vi "RunVis.vi"(6 "Re-Init":bool, 7 "Index":i8, 8 "dt":i8, 9 "HMI to Control":T1, 10 "SensorInputData":T5, 11 "arguments":string[](array[string])) -> (1 "Done":bool, 2 "HMI to Control Out":T1, 3 "SensorInputDataOut":T5)   [LabVIEW 2015]
uses:
  Typedefs/Arm States.ctl
  Typedefs/IntakeWheelSenseOrManual.ctl
  Typedefs/ClawStates.ctl
  Typedefs/HMI_to_Control.ctl
  Typedefs/SensorInputData.ctl
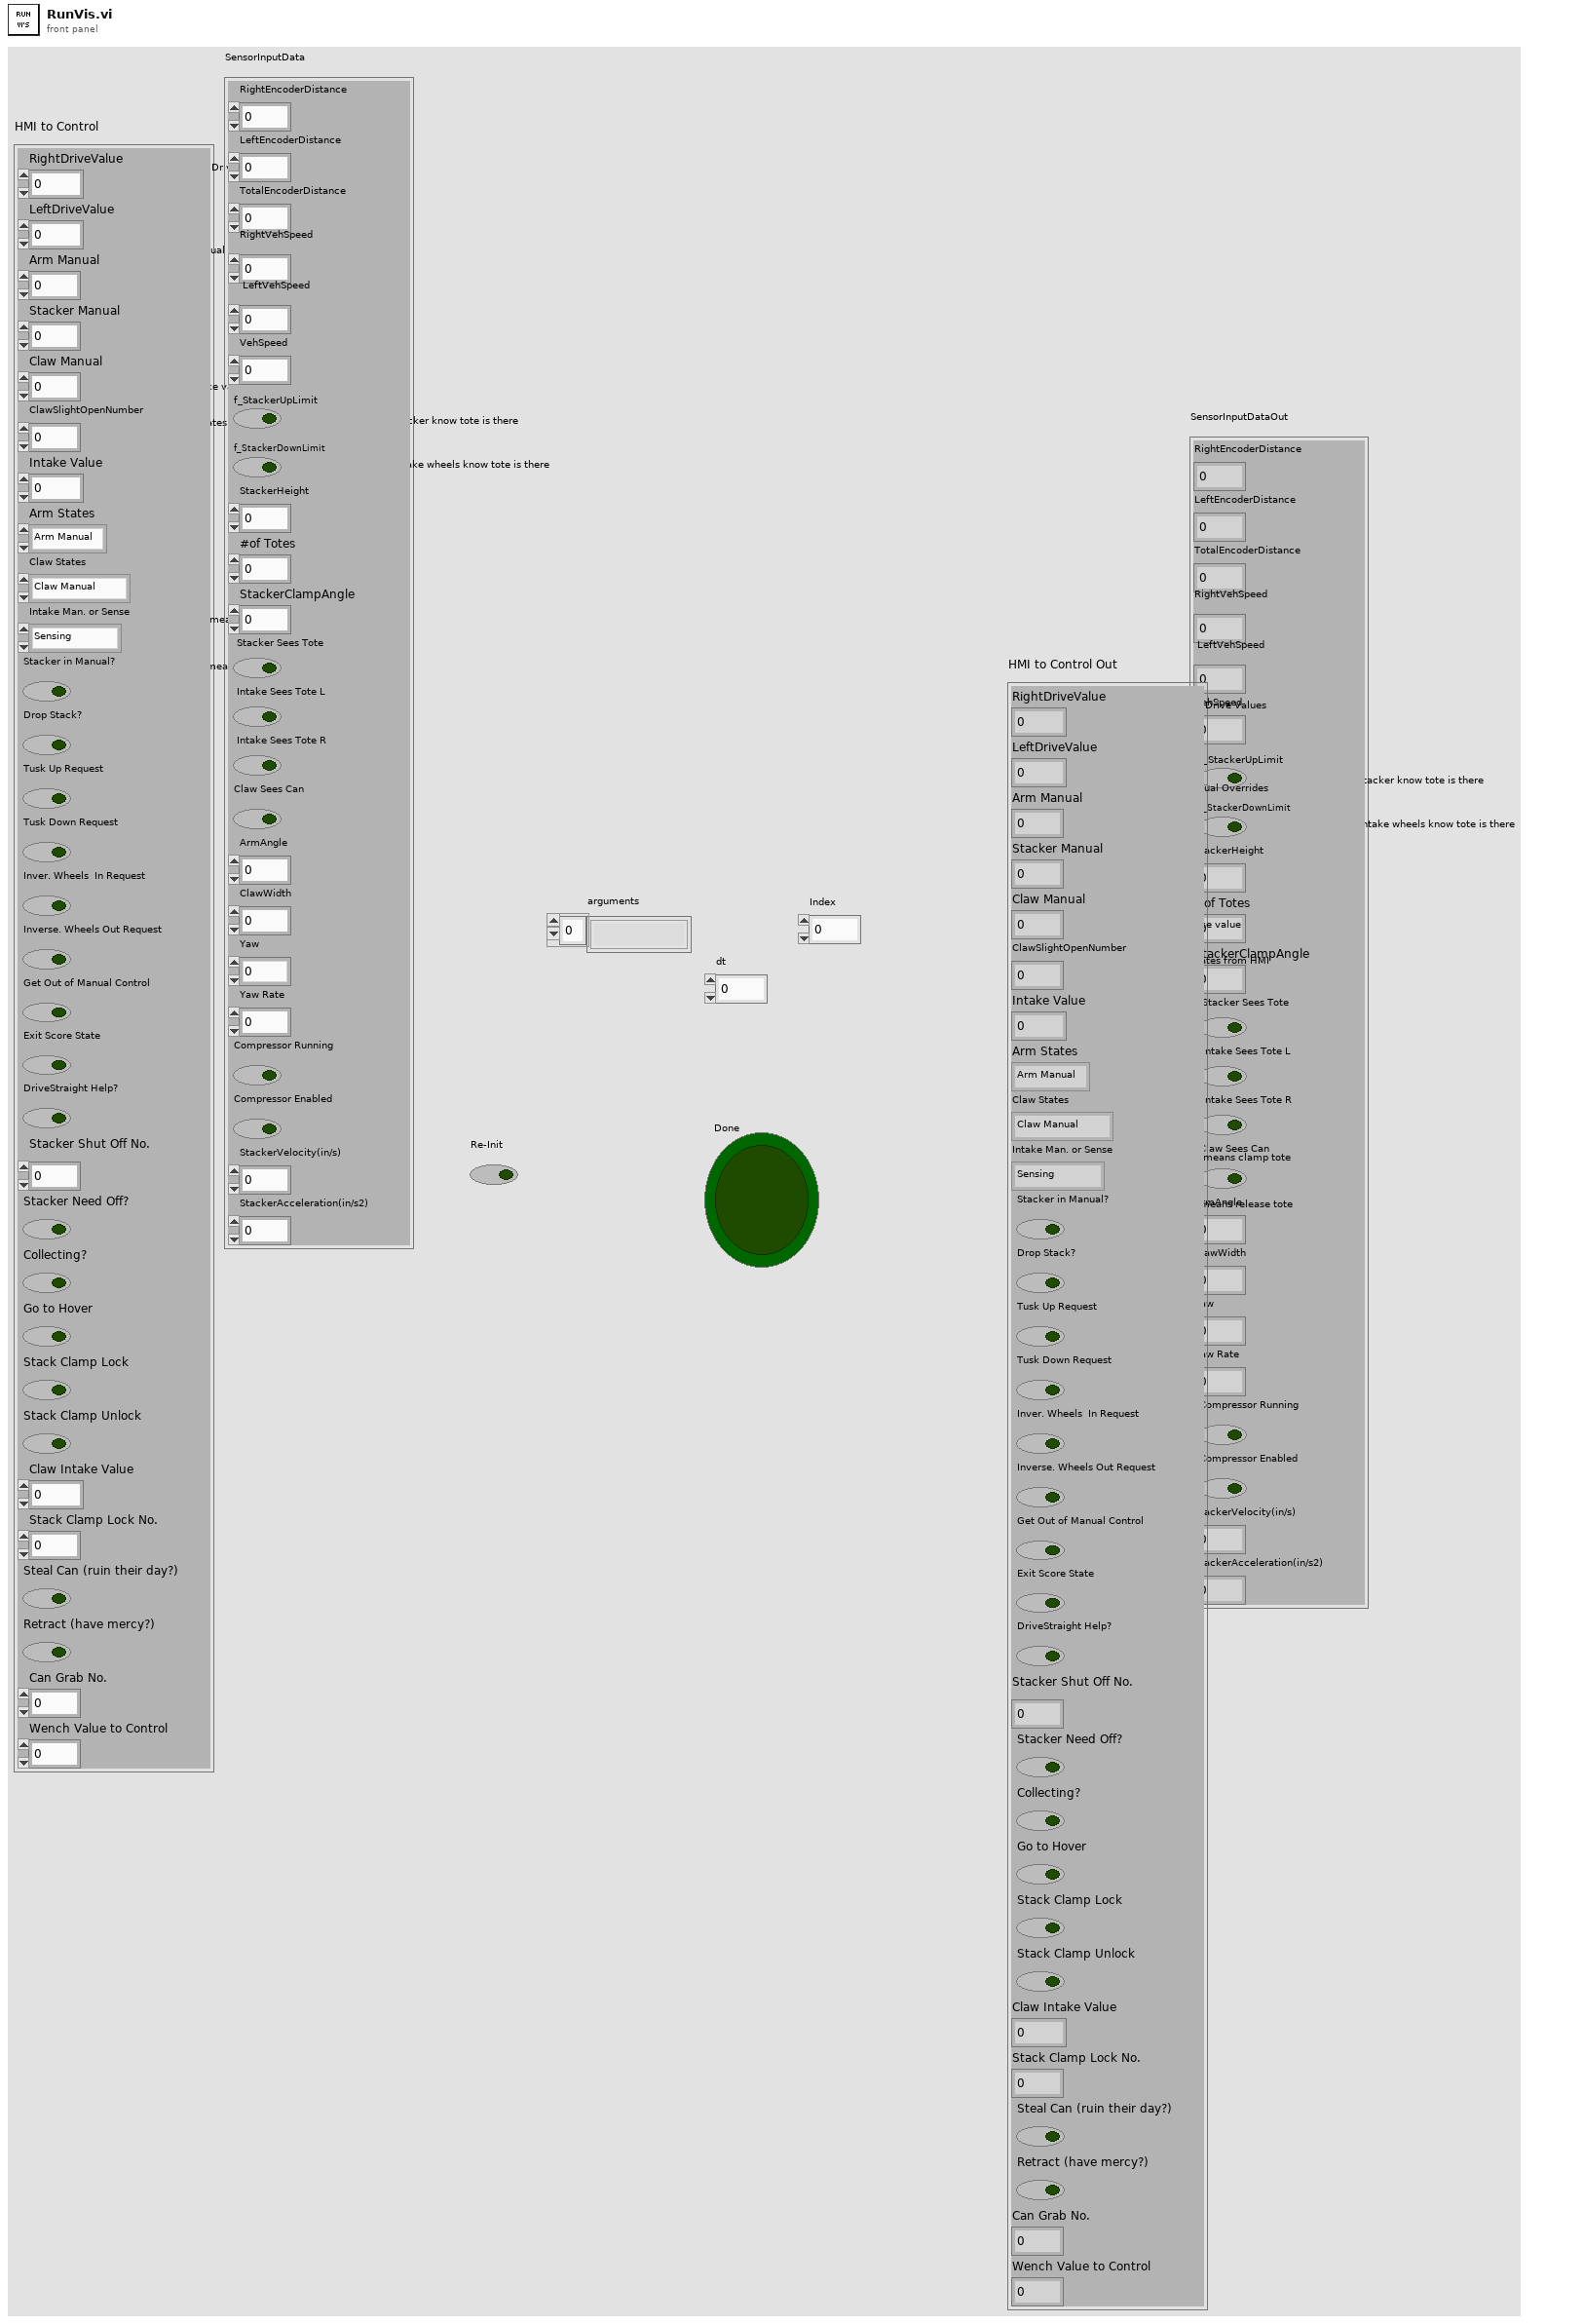
[diagram p1: front panel]
types:
  T1 = typedef "HMI_to_Control.ctl" = cluster{"RightDriveValue":dbl, "LeftDriveValue":dbl, "Arm Manual ":dbl, "Stacker Manual ":dbl, "Claw Manual ":dbl, "ClawSlightOpenNumber":i8, "Intake Value ":sgl, "Arm States":T2, "Claw States":T3, "Intake Man. or Sense":T4, "Stacker in Manual?":bool, "Drop Stack? ":bool, "Tusk Up Request":bool, "Tusk Down Request":bool, "Inver. Wheels  In Request":bool, "Inverse. Wheels Out Request ":bool, "Get Out of Manual Control":bool, "Exit Score State":bool, "DriveStraight Help?":bool, "Stacker Shut Off No.":i8, "Stacker Need Off?":bool, "Collecting?":bool, "Go to Hover":bool, "Stack Clamp Lock ":bool, "Stack Clamp Unlock ":bool, "Claw Intake Value ":sgl, "Stack Clamp Lock No. ":i8, "Steal Can (ruin their day?)":bool, "Retract (have mercy?)":bool, "Can Grab No. ":i8, "Wench Value to Control ":dbl}
  T2 = typedef "Arm States.ctl" = enum16{"Arm Manual ", "Ground", "Step", "1 Tote", "2 Tote", "3 Tote", "4 Tote", "5 Tote", "6 Tote", "Flip Can Arm", "Grab Can in auto", "Nudge"}
  T3 = typedef "ClawStates.ctl" = enum16{"Claw Manual ", "Claw Open", "Claw Closed", "Claw Slight Open", "Flip Can"}
  T4 = typedef "IntakeWheelSenseOrManual.ctl" = enum16{"Sensing", "Manual "}
  T5 = typedef "SensorInputData.ctl" = cluster{"RightEncoderDistance":dbl, "LeftEncoderDistance":dbl, "TotalEncoderDistance":dbl, "RightVehSpeed":dbl, "LeftVehSpeed":dbl, "VehSpeed":dbl, "f_StackerUpLimit":bool, "f_StackerDownLimit":bool, "StackerHeight":dbl, "#of Totes":u8, "StackerClampAngle":dbl, "Stacker Sees Tote":bool, "Intake Sees Tote L":bool, "Intake Sees Tote R":bool, "Claw Sees Can":bool, "ArmAngle":dbl, "ClawWidth":dbl, "Yaw":dbl, "Yaw Rate":dbl, "Compressor Running":bool, "Compressor Enabled":bool, "StackerVelocity(in/s)":dbl, "StackerAcceleration(in/s2)":dbl}
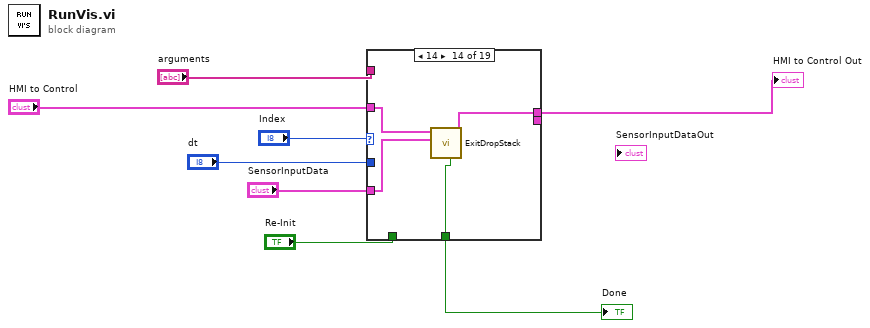
[diagram p0: block diagram]
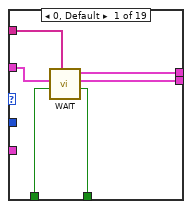
[diagram p2: hidden frame]
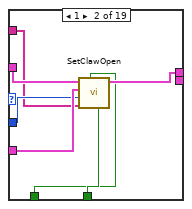
[diagram p3: hidden frame]
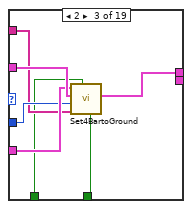
[diagram p4: hidden frame]
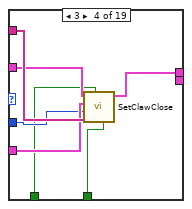
[diagram p5: hidden frame]
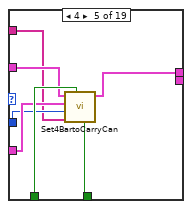
[diagram p6: hidden frame]
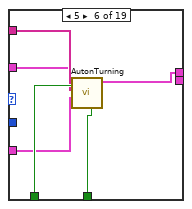
[diagram p7: hidden frame]
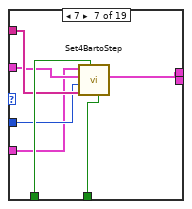
[diagram p8: hidden frame]
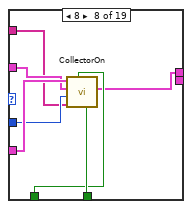
[diagram p9: hidden frame]
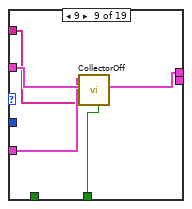
[diagram p10: hidden frame]
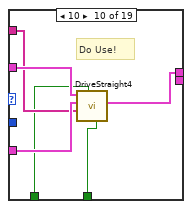
[diagram p11: hidden frame]
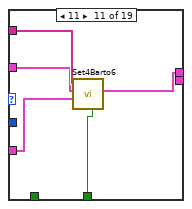
[diagram p12: hidden frame]
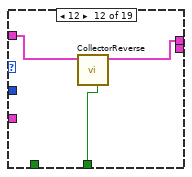
[diagram p13: hidden frame]
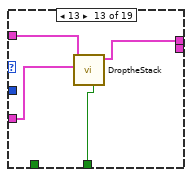
[diagram p14: hidden frame]
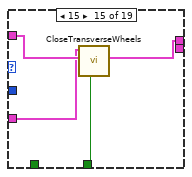
[diagram p15: hidden frame]
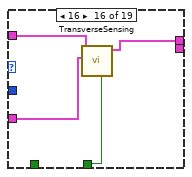
[diagram p16: hidden frame]
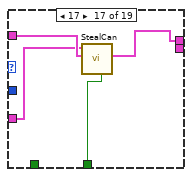
[diagram p17: hidden frame]
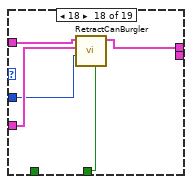
[diagram p18: hidden frame]
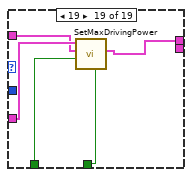
[diagram p19: hidden frame]
diagram:
  n1 = case shown="14" "Index" {
    tunnel: "HMI to Control" -> [w12 w20 w28 w34 w40 w44 w51 w59 w66 w73 w77 w80 w84 w89 w93 w97 w100 w104 w108]
    tunnel: "SensorInputData" -> [_ w19 w27 w33 w39 w45 w50 w60 w65 w72 w76 _ w83 w88 w92 w96 w99 w103 w109]
    tunnel: [w14 w21 w25 w30 w41 w47 w55 w62 w67 w69 w75 w81 w85 w87 w91 w95 w101 w106 w111] -> w5
    tunnel: "Re-Init" -> [w9 w16 w22 w31 w42 w48 w54 w61 _ w70 _ _ _ _ _ _ _ _ w110]
    tunnel: "arguments" -> [w13 w15 w23 w35 w37 w46 w53 w57 w64 w71 w78 _ _ _ _ _ _ _ _]
    tunnel: "dt" -> [_ w18 w24 w32 w38 _ w52 w58 _ _ _ _ _ _ _ _ _ w102 _]
    tunnel: [w11 w17 w26 w29 w36 w43 w49 w56 w63 w68 w74 w79 w82 w86 w90 w94 w98 w105 w107] -> w1
    tunnel: [w10 _ _ _ _ _ _ _ _ _ _ _ _ _ _ _ _ _ _] -> _
    frame 0, Default {
      n2 = call "WAIT.vi"("arguments"=w13, "Reinit"=w9, "HMI to Control"=w12) -> ("Done"=w14:bool, "SensorInputDataOut"=w10:T5, "HMI to Control Out"=w11:T1)  [unwired: 6 in]
    }
    frame 1 {
      n3 = call "SetClawOpen.vi"("Reinit"=w16, "arguments"=w15, "dt"=w18, "SensorInputData"=w19, "HMI to Control"=w20) -> ("HMI to ControlOut"=w17:T1, "Done"=w21:bool)  [unwired: 4 in, 1 out]
    }
    frame 2 {
      n4 = call "Set4BartoGround.vi"("Reinit"=w22, "arguments"=w23, "dt"=w24, "HMI to Control"=w28, "SensorInputData"=w27) -> ("HMI to ControlOut"=w26:T1, "Done"=w25:bool)  [unwired: 4 in, 1 out]
    }
    frame 3 {
      n5 = call "SetClawClose.vi"("Reinit"=w31, "arguments"=w35, "dt"=w32, "SensorInputData"=w33, "HMI to Control"=w34) -> ("HMI to ControlOut"=w29:T1, "Done"=w30:bool)  [unwired: 4 in, 1 out]
    }
    frame 4 {
      n6 = call "Set4BartoCarryCan.vi"("Reinit"=w42, "arguments"=w37, "dt"=w38, "SensorInputData"=w39, "HMI to Control"=w40) -> ("HMI to ControlOut"=w36:T1, "Done"=w41:bool)  [unwired: 4 in, 1 out]
    }
    frame 5 {
      n7 = call "AutonTurning.vi"("Re-Init"=w48, "SensorInputData"=w45, "arguments"=w46, "HMI to Control"=w44) -> ("HMI to Control Out"=w43:T1, "Done"=w47:bool)  [unwired: 5 in, 1 out]
    }
    frame 7 {
      n8 = call "Set4BartoStep.vi"("Reinit"=w54, "arguments"=w53, "dt"=w52, "HMI to Control"=w51, "SensorInputData"=w50) -> ("HMI to ControlOut"=w49:T1, "Done"=w55:bool)  [unwired: 4 in, 1 out]
    }
    frame 8 {
      n9 = call "CollectorOn.vi"("Reinit"=w61, "arguments"=w57, "dt"=w58, "HMI to Control"=w59, "SensorInputData"=w60) -> ("HMI to ControlOut"=w56:T1, "Done"=w62:bool)  [unwired: 4 in, 1 out]
    }
    frame 9 {
      n10 = call "CollectorOff.vi"("arguments"=w64, "HMI to Control"=w66, "SensorInputData"=w65) -> ("HMI to ControlOut"=w63:T1, "Done"=w67:bool)  [unwired: 6 in, 1 out]
    }
    frame 10 {
      # "Do Use!"
      n11 = call "DriveStraight4.vi"("Re-Init"=w70, "arguments"=w71, "SensorInputData"=w72, "HMI to Control"=w73) -> ("HMI to Control Out"=w68:T1, "Done"=w69:bool)  [unwired: 5 in, 1 out]
    }
    frame 11 {
      n12 = call "Set4Barto6.vi"("SensorInputData"=w76, "HMI to Control"=w77, "arguments"=w78) -> ("HMI to ControlOut"=w74:T1, "Done"=w75:bool)  [unwired: 6 in, 1 out]
    }
    frame 12 {
      n13 = call "CollectorReverse.vi"("HMI to Control"=w80) -> ("HMI to ControlOut"=w79:T1, "Done"=w81:bool)  [unwired: 9 in]
    }
    frame 13 {
      n14 = call "DroptheStack.vi"("SensorInputData"=w83, "HMI to Control"=w84) -> ("HMI to ControlOut"=w82:T1, "Done"=w85:bool)  [unwired: 7 in, 1 out]
    }
    frame 14 {
      n15 = call "ExitDropStack.vi"("SensorInputData"=w88, "HMI to Control"=w89) -> ("HMI to ControlOut"=w86:T1, "Done"=w87:bool)  [unwired: 7 in, 1 out]
    }
    frame 15 {
      n16 = call "CloseTransverseWheels.vi"("HMI to Control"=w93, "SensorInputData"=w92) -> ("HMI to ControlOut"=w90:T1, "Done"=w91:bool)  [unwired: 7 in, 1 out]
    }
    frame 16 {
      n17 = call "TransverseSensing.vi"("SensorInputData"=w96, "HMI to Control"=w97) -> ("HMI to ControlOut"=w94:T1, "Done"=w95:bool)  [unwired: 7 in, 1 out]
    }
    frame 17 {
      n18 = call "StealCan.vi"("HMI to Control"=w100, "SensorInputData"=w99) -> ("HMI to ControlOut"=w98:T1, "Done"=w101:bool)  [unwired: 7 in, 1 out]
    }
    frame 18 {
      n19 = call "RetractCanBurgler.vi"("dt"=w102, "SensorInputData"=w103, "HMI to Control"=w104) -> ("HMI to ControlOut"=w105:T1, "Done"=w106:bool)  [unwired: 6 in, 1 out]
    }
    frame 19 {
      n20 = call "SetMaxDrivingPower.vi"("Reinit"=w110, "HMI to Control"=w108, "SensorInputData"=w109) -> ("HMI to ControlOut"=w107:T1, "Done"=w111:bool)  [unwired: 6 in, 1 out]
    }
  }
  "HMI to Control Out" <- w1
  "Done" <- w5
